vi "Calibrate Acoustic Output Level.vi"() -> ()   [LabVIEW 2022 SP3]
uses:
  <vilib>/addons/_NISVFA/_Generation/Signal Generation/SV Signal/sv_System Timing Model.ctl
  <vilib>/Analysis/1siggen.llb/Ramp Pattern by Samples.vi
  <vilib>/DAQmx/write.llb/DAQmx Write (Analog Wfm 1Chan NSamp).vi
  <vilib>/DAQmx/read.llb/DAQmx Read (Analog Wfm 1Chan NSamp).vi
  <vilib>/addons/_NISVFA/_Generation/Signal Generation/SV Sinusoid/SV Sinusoid.lvclass
  C:/Program Files/NI/LVAddons/nisvt/1/vi.lib/addons/_NISVFA/_Generation/Signal Generation/SV Signal/SV Signal.lvclass
  <vilib>/addons/_NISVFA/_Generation/Signal Generation/SV Sinusoid/Configure Sine.vi
  <vilib>/DAQmx/create/channels.llb/DAQmx Create Channel (AO-Voltage-Basic).vi
  <vilib>/DAQmx/configure/timing.llb/DAQmx Timing (Sample Clock).vi
  <vilib>/DAQmx/create/channels.llb/DAQmx Create Channel (AI-Sound Pressure-Microphone).vi
  <vilib>/addons/_NISVFA/_Generation/Signal Generation/SV Signal/Write Sample Rate.vi
  <vilib>/addons/_NISVFA/_Generation/Signal Generation/SV Signal/Write System Timing Model.vi
  <vilib>/addons/_NISVFA/_Generation/Signal Generation/SV Signal/Write Ramp Parameters.vi
  <vilib>/DAQmx/miscellaneous.llb/DAQmx Fill In Error Info.vi
  <vilib>/addons/Sound and Vibration/svt_Level/SVL Leq Sound Level (1 Ch).vi
  <vilib>/addons/_NISVFA/_Generation/Signal Generation/SV Signal/SV Signal.lvclass
  <resource>/objmgr/daqmx.rc
  <vilib>/Analysis/NI_AALBase.lvlib
  <vilib>/addons/Sound and Vibration/svt_Level/SoundVib_SoundLevel.lvlib
  <vilib>/gmath/NI_Gmath.lvlib
  C:/Program Files/NI/LVAddons/nisvt/1/vi.lib/addons/_NISVFA/_Generation/Signal Generation/SV Function/SV Function.lvclass
  C:/Program Files/NI/LVAddons/nisvt/1/vi.lib/addons/_NISVFA/_Generation/Signal Generation/SV Sinusoid/SV Sinusoid.lvclass
panel:
  out "crossed":bool
  out "output voltage ratio":dbl format="%#_g Pa/Vpk"
  in  "target value":dbl=80.0 format="%#_g dB"
  in  "number of steps":dbl=4.0
  in  "stop amplitude":dbl=1.0 format="%#_g Vpk"
  out "dBSPL":dbl=82.82326800651335
  out "Waveform Graph":waveform(dbl)(graph)={"t0"=timestamp(3812031326.7400646 s since 1904-01-01), "dt"=1.9531249997269942e-05, "Y"=array[5120 elements], "attributes"=variant("NI_ChannelName"=variant(string "PXI1Slot2/ai0"), "NI_UnitDescription"=variant(string "Pascals"), "NI_dBReference"=variant(dbl 2e-05))}
  in  "sensor sensitivity [mV/Pa]":dbl=50.0
  in  "physical channel":tag="PXI1Slot2/ai0"
  in  "output channels":tag="PXI1Slot2/ao0"
  in  "start amplitude":dbl=0.1 format="%#_g Vpk"
  in  "frequency":dbl=1000.0 format="%#_g Hz"
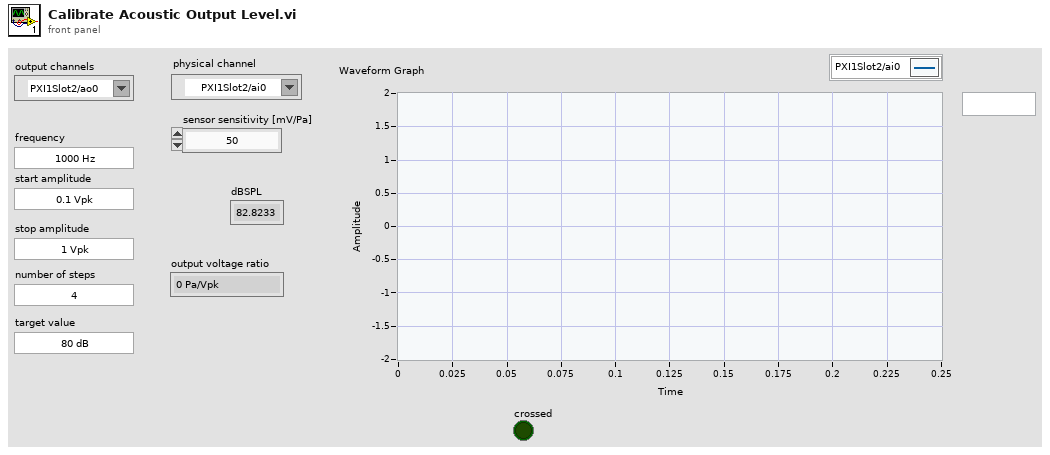
[diagram p1: front panel]
types:
  T1 = typedef "SV Signal.lvclass/sv_System Timing Model.ctl" = i64
  T2 = cluster{"profile":enum16{"Linear", "Half cosine"}, "durations [s]":cluster{"ramp-up":dbl, "transition":dbl, "ramp-down":dbl}}
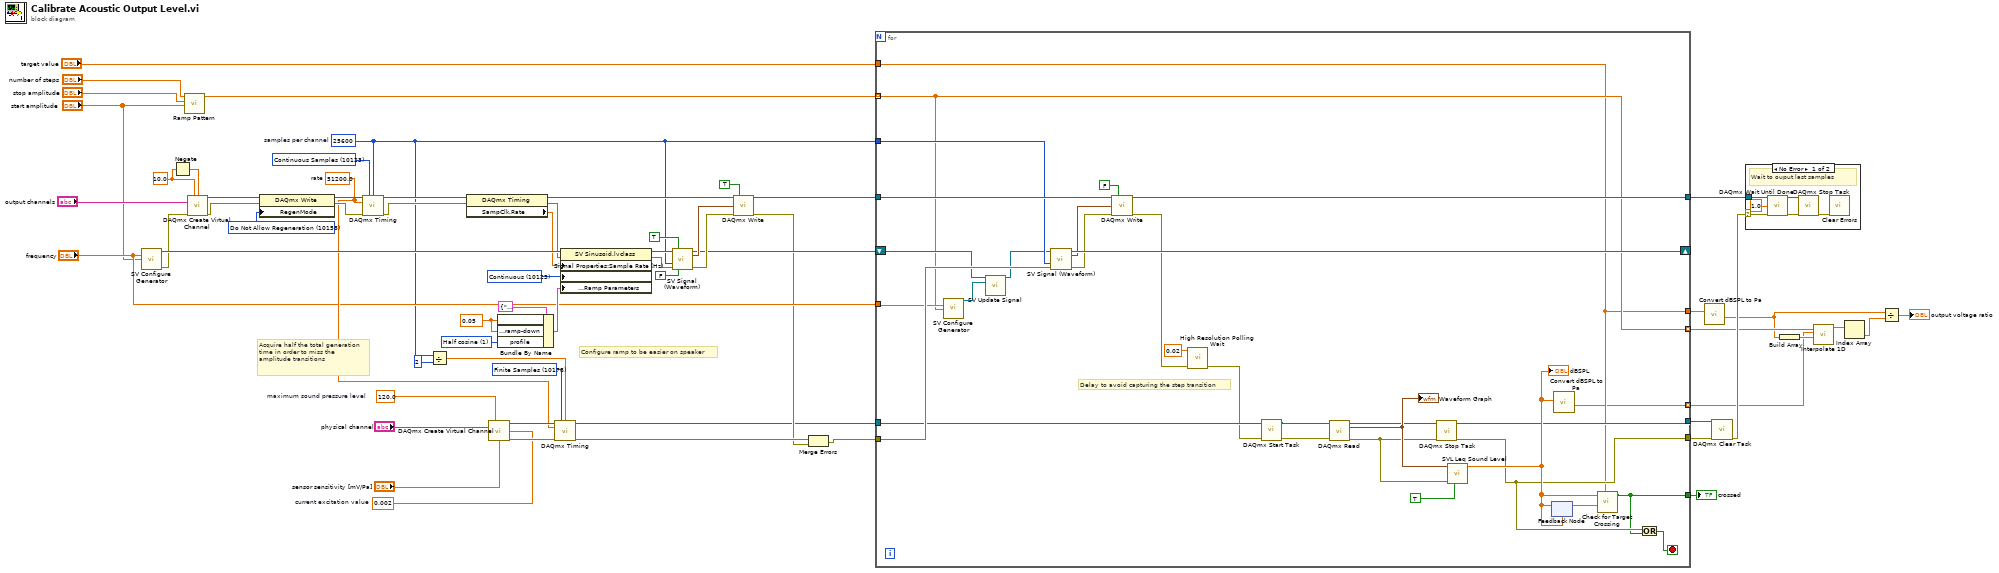
[diagram p0: block diagram]
diagram:
  w62 = 0.05 ("ramp duration")
  w60 = u16 1 items=["Linear", "Half cosine"] ("ramp profile")
  w37 = 0.002  # current excitation value
  w41 = 120.0  # maximum sound pressure level
  w43 = 10178 items=["Finite Samples"=10178, "Continuous Samples"=10123] ("sample mode")
  w50 = 10158 items=["Allow Regeneration"=10097, "Do Not Allow Regeneration"=10158] ("RegenMode")
  w54 = 10.0 ("maximum value")
  w14 = 25600  # samples per channel
  w56 = 10123 items=["Finite Samples"=10178, "Continuous Samples"=10123, "Hardware Timed Single Point"=12522] ("sample mode")
  w23 = 51200.0  # rate
  w59 = T1 10123 items=["Finite"=10178, "-"=-1, "Continuous"=10123, "-"=-2, "Settled"=110123, "Averaged"=210123, "Discrete Sweep"=310123, "Continuous Sweep"=410123] ("System Timing Model")
  # "Acquire half the total generation time in order to miss the amplitude transitions"
  # "Configure ramp to be easier on speaker"
  n1 = call-poly <vilib>:"SV Configure Generator.vi"("frequency (Hz)"="frequency", "amplitude"="start amplitude") -> ("signal configuration"=w64:refnum<class "SV Sinusoid.lvclass">, "error out"=w52:errorcluster)  [unwired: 12 in]
  n2 = Negate(x=w54) -> (-x=w53:dbl)
  n3 = call-poly <vilib>:"Ramp Pattern.vi"("start"="start amplitude", "end"="stop amplitude", "samples"="number of steps") -> ("Ramp Pattern"=w19:dbl[])  [unwired: 7 in, 1 out]
  n4 = call-poly <vilib>:"DAQmx Create Virtual Channel.vi"("maximum value"=w54, "minimum value"=w53, "physical channels"="output channels", "error in"=w52) -> ("task out"=w49:refnum<k21>, "error out"=w47:errorcluster)  [unwired: 10 in]
  n5 = property class="DAQmx Write"(reference=w49, error in=w47, "RegenMode"=w50) -> (reference out=w48:refnum<k21>, error out=w46:errorcluster)
  n6 = call-poly <vilib>:"DAQmx Timing.vi"("task/channels in"=w48, "sample mode"=w56, "samples per channel"=w14, "rate"=w23, "error in"=w46) -> ("task out"=w57:refnum<k21>, "error out"=w55:errorcluster)  [unwired: 9 in]
  n7 = Divide(x=w14, y=2) -> (x/y=w12:dbl)
  n8 = property class="DAQmx Timing"(reference=w57, error in=w55) -> (reference out=w34:refnum<k21>, error out=w44:errorcluster, "SampClk.Rate"=w45:dbl)
  n9 = call-poly <vilib>:"DAQmx Create Virtual Channel.vi"("maximum sound pressure level"=w41, "physical channels"="physical channel", "current excitation value"=w37, "microphone sensitivity"="sensor sensitivity [mV/Pa]") -> ("task out"=w39:refnum<k21>, "error out"=w38:errorcluster)  [unwired: 10 in]
  n10 = Bundle By Name(cluster=T2 {"profile"=enum."Linear", "durations [s]"={"ramp-up"=0.0, "transition"=0.0, "ramp-down"=0.0}} ("Ramp Parameters:All Elements"), "durations [s].ramp-up"=w62, "durations [s].ramp-down"=w62, "profile"=w60) -> (w61:T2)
  n11 = call-poly <vilib>:"DAQmx Timing.vi"("task/channels in"=w39, "sample mode"=w43, "samples per channel"=w12, "rate"=w23, "error in"=w38) -> ("task out"=w16:refnum<k21>, "error out"=w26:errorcluster)  [unwired: 9 in]
  n12 = property class="SV Sinusoid.lvclass"(reference=w64, error in=w44, "Signal Properties:Sample Rate (Hz)"=w45, "Signal Properties:System Timing Model"=w59, "Signal Properties:Ramps:Ramp Parameters"=w61) -> (reference out=w33:refnum<class "SV Sinusoid.lvclass">, error out=w32:errorcluster)
  n13 = call-dynamic "SV Signal (Waveform).vi"("signal configuration"=w33, "reset"=TRUE, "samples"=w14, "error in (no error)"=w32, "stop"=FALSE) -> ("signal configuration"=w27:refnum<class "SV Sinusoid.lvclass">, "output waveform"=w35:waveform(dbl), "error out"=w36:errorcluster)  [unwired: 5 in, 3 out]
  n14 = call-poly <vilib>:"DAQmx Write.vi"("task/channels in"=w34, "auto start"=TRUE, "data"=w35, "error in"=w36) -> ("task out"=w30:refnum<k21>, "error out"=w17:errorcluster)  [unwired: 9 in, 1 out]
  n15 = Merge Errors(w26, w17) -> (w15:errorcluster)
  n16 = for {
    shift-right: [w95] -> _
    shift-left: w27 -> [w86]
    tunnel: w14 -> [w89]
    tunnel: w30 -> [w94]
    tunnel: [w93] -> w51
    tunnel: w15 -> [w88]
    tunnel: w16 -> [w78]
    tunnel: [w73] -> w25
    tunnel: "frequency" -> [w84]
    tunnel: [w72] -> w21
    tunnel: w19 -> [w67] mode=indexing
    tunnel: "target value" -> [w66]
    tunnel: [w68] -> w2
    tunnel: [w67] -> w5 mode=indexing
    tunnel: [w65] -> w10 mode=indexing
    tunnel: [w66] -> w9
    stop <- w82 stop-if-true
    # "Delay to avoid capturing the step transition"
    n17 = call-poly <vilib>:"SV Configure Generator.vi"("frequency (Hz)"=w84, "amplitude"=w67) -> ("signal configuration"=w87:refnum<class "SV Sinusoid.lvclass">)  [unwired: 12 in, 1 out]
    n18 = call-dynamic "SV Update Signal.vi"("current configuration"=w86, "new configuration"=w87) -> ("updated configuration"=w85:refnum<class "SV Sinusoid.lvclass">)  [unwired: 12 in, 1 out]
    n19 = call-dynamic "SV Signal (Waveform).vi"("signal configuration"=w85, "samples"=w89, "error in (no error)"=w88) -> ("signal configuration"=w95:refnum<class "SV Sinusoid.lvclass">, "output waveform"=w90:waveform(dbl), "error out"=w92:errorcluster)  [unwired: 7 in, 3 out]
    n20 = call-poly <vilib>:"DAQmx Write.vi"("task/channels in"=w94, "auto start"=FALSE, "data"=w90, "error in"=w92) -> ("task out"=w93:refnum<k21>, "error out"=w71:errorcluster)  [unwired: 9 in, 1 out]
    n21 = call <vilib>:"High Resolution Polling Wait.vi"("error in (no error)"=w71, "seconds to wait"=0.02) -> ("error out"=w70:errorcluster)  [unwired: 9 in]
    n22 = call <vilib>:"DAQmx Start Task.vi"("task/channels in"=w78, "error in"=w70) -> ("task out"=w77:refnum<k21>, "error out"=w76:errorcluster)  [unwired: 12 in]
    n23 = call-poly <vilib>:"DAQmx Read.vi"("task/channels in"=w77, "error in"=w76) -> ("task out"=w75:refnum<k21>, "data"=w79:waveform(dbl), "error out"=w74:errorcluster)  [unwired: 11 in]
    "Waveform Graph" <- w79
    n24 = call <vilib>:"DAQmx Stop Task.vi"("task/channels in"=w75, "error in"=w74) -> ("task out"=w73:refnum<k21>, "error out"=w72:errorcluster)  [unwired: 12 in]
    n25 = call-poly <vilib>:"SVL Leq Sound Level.vi"("restart averaging (F)"=TRUE, "error in (no error)"=w74, "scaled signal [EU]"=w79) -> ("Leq sound level [dB EU]"=w80:dbl)  [unwired: 6 in, 2 out]
    "dBSPL" <- w80
    n26 = feedback-in #1(w80) -> ()
    n27 = feedback #1(w80) -> (w81:dbl)
    n28 = call "Convert dBSPL to Pa.vi"("dB SPL"=w80) -> ("Pa pk"=w65:dbl)  [unwired: 9 in, 1 out]
    n29 = call "Check for Target Crossing.vi"("target value"=w66, "previous value"=w81, "current value"=w80) -> ("crossed"=w68:bool)  [unwired: 8 in]
    n30 = Or(x=w72, y=w68) -> (x .or. y?=w82:bool)
  }
  "crossed" <- w2
  n31 = call "Convert dBSPL to Pa.vi"("dB SPL"=w9) -> ("Pa pk"=w1:dbl)  [unwired: 9 in, 1 out]
  n32 = call <vilib>:"DAQmx Clear Task.vi"("task in"=w25, "error in"=w21) -> ("error out"=w24:errorcluster)  [unwired: 13 in]
  n33 = case shown="No Error" w24 {
    selector: w24 -> [w98 _]
    tunnel: w51 -> [w101 _]
    frame No Error {
      # "Wait to ouput last samples"
      n34 = call <vilib>:"DAQmx Wait Until Done.vi"("task/channels in"=w101, "timeout (sec)"=1.0, "error in"=w98) -> ("task out"=w100:refnum<k21>, "error out"=w99:errorcluster)  [unwired: 11 in]
      n35 = call <vilib>:"DAQmx Stop Task.vi"("task/channels in"=w100, "error in"=w99) -> ("error out"=w97:errorcluster)  [unwired: 12 in, 1 out]
      n36 = call <vilib>:"Clear Errors.vi"("error in (no error)"=w97) -> ()  [unwired: 5 in, 2 out]
    }
    frame Error {
      # "Error"
    }
  }
  n37 = Build Array(w1) -> (w11:dbl[])
  n38 = call <vilib>:"Interpolate 1D.vi"("xi"=w11, "X"=w10, "Y"=w5) -> ("yi"=w8:dbl[])  [unwired: 6 in, 2 out]
  n39 = Index Array(array=w8) -> (element=w7:dbl)  [unwired: 1 in]
  n40 = Divide(x=w1, y=w7) -> (x/y=→"output voltage ratio":dbl)
